vi "Move.vi"(9 "Direction":T1, 11 "Cross.lvclass":refnum<class "Cross.lvclass">) -> (1 "Direction 2":T1, 3 "Cross.lvclass 2":refnum<class "Cross.lvclass">)   [LabVIEW 2015, in "Cross.lvclass"]
uses:
  Cross.lvclass
  Type Defs/Direction Enum.ctl
  Cross.lvclass/Cross.ctl
  Type Defs/SB Type Defs.lvlib
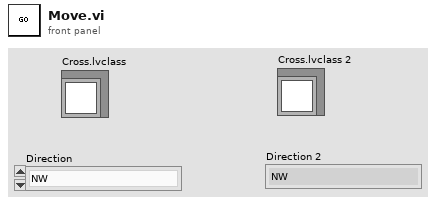
[diagram p1: front panel]
types:
  T1 = typedef "SB Type Defs.lvlib/Direction Enum.ctl" = enum16{"NW", "N", "NE", "E", "SE", "S", "SW", "W"}
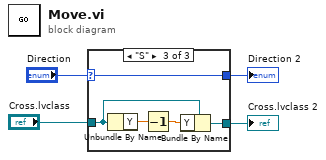
[diagram p0: block diagram]
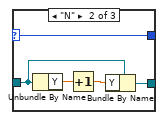
[diagram p3: hidden frame]
diagram:
  n1 = case shown="\"S\"" "Direction" {
    selector: "Direction" -> [w6 w11 w16]
    tunnel: [w6 w11 w16] -> w3
    tunnel: "Cross.lvclass" -> [w5 w10 w15]
    tunnel: [w5 w9 w14] -> w1
    frame "NW", Default {
    }
    frame "N" {
      n2 = Unbundle By Name(w10) -> ("Y"=w8:dbl)
      n3 = Increment(x=w8) -> (x+1=w7:dbl)
      n4 = Bundle By Name(cluster=w10, "Y"=w7) -> (w9:refnum<class "Cross.lvclass">)
    }
    frame "S" {
      n5 = Unbundle By Name(w15) -> ("Y"=w13:dbl)
      n6 = Decrement(x=w13) -> (x-1=w12:dbl)
      n7 = Bundle By Name(cluster=w15, "Y"=w12) -> (w14:refnum<class "Cross.lvclass">)
    }
  }
  "Cross.lvclass 2" <- w1
  "Direction 2" <- w3
